vi "JSON GRUPO 2.vi"(8 "error in":errorcluster, 11 "Grupo in":T1(array[cluster])) -> (0 "error out":errorcluster, 1 "alarmas":refnum<class "JSON Array.lvclass">[](array[class]), 2 "JSON BAT":refnum<class "JSON Object.lvclass">[](array[class]), 3 "JSON CARGA":refnum<class "JSON Array.lvclass">[](array[class]), 5 "JSON FV":refnum<class "JSON Object.lvclass">[](array[class]))   [LabVIEW 2015]
uses:
  <vilib>/addons/JSON API/JSON Scalar/Set SGL.vi
  <vilib>/addons/JSON API/JSON Scalar/Set U32.vi
  <vilib>/addons/JSON API/JSON Object/JSON Object.lvclass
  <vilib>/addons/JSON API/JSON Array/JSON Array.lvclass
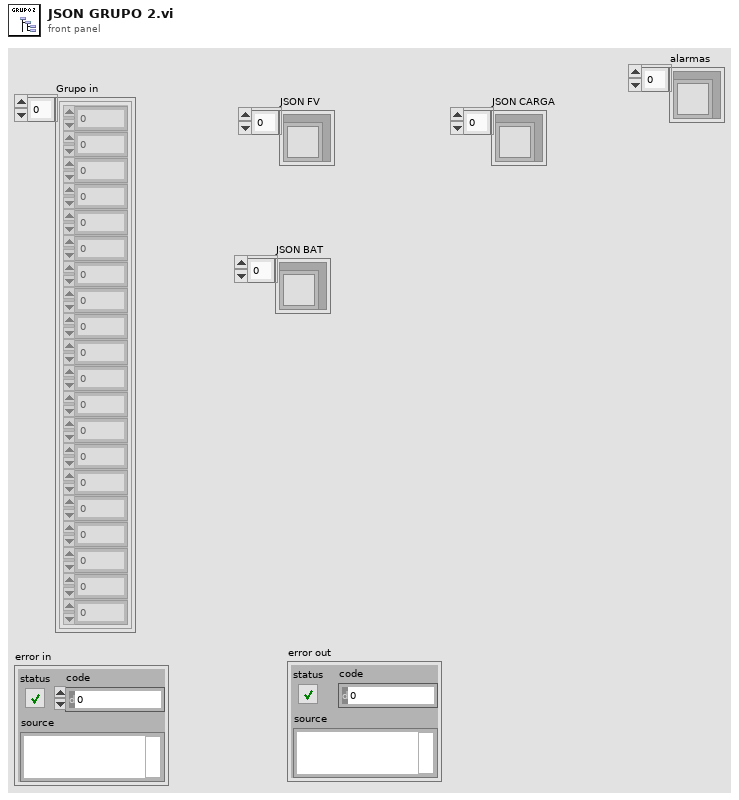
[diagram p1: front panel]
types:
  T1 = cluster{u32, dbl, dbl, dbl, dbl, dbl, dbl, dbl, dbl, dbl, dbl, dbl, dbl, dbl, dbl, dbl, dbl, dbl, dbl, dbl}[]
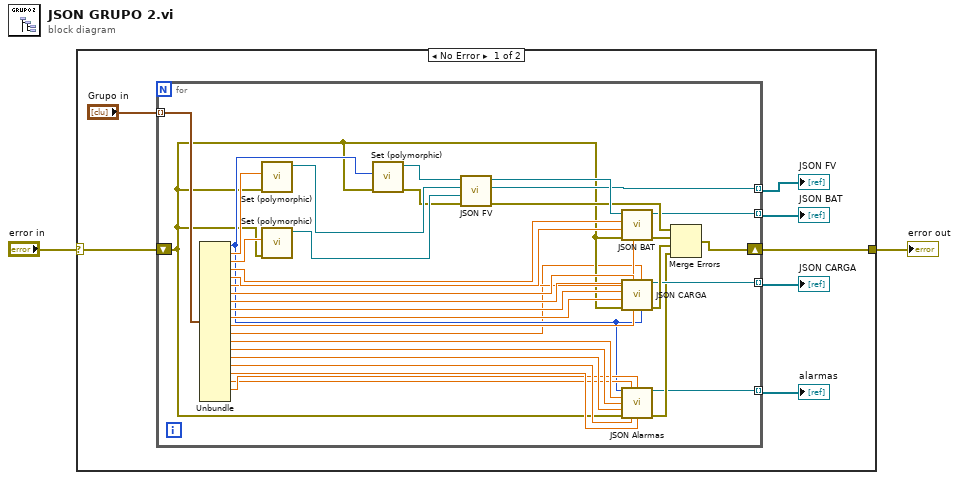
[diagram p0: block diagram]
diagram:
  n1 = case shown="No Error" "error in" {
    selector: "error in" -> [w3 w45]
    tunnel: [w4 w45] -> w1
    frame No Error {
      n2 = for {
        tunnel: "Grupo in" -> [w44] mode=indexing
        tunnel: [w28] -> w6 mode=indexing
        tunnel: [w27] -> w7 mode=indexing
        tunnel: [w26] -> w8 mode=indexing
        tunnel: [w13] -> w5 mode=indexing
        shift-right: [w12] -> w4
        shift-left: w3 -> [w11]
        n3 = Unbundle(w44) -> (w15:u32, w42:dbl, w41:dbl, w40:dbl, w37:dbl, w32:dbl, w34:dbl, w33:dbl, w25:dbl, w24:dbl, w23:dbl, w10:dbl, w22:dbl, w21:dbl, w20:dbl, w19:dbl, w18:dbl, w16:dbl, w17:dbl)  [unwired: 1 out]
        n4 = call-poly <vilib>:"Set (polymorphic).vi"("error in (no error)"=w11, "Numeric"=w42) -> ("JSON Scalar out"=w39:refnum<class "JSON Scalar.lvclass">)  [unwired: 8 in, 1 out]
        n5 = call-poly <vilib>:"Set (polymorphic).vi"("error in (no error)"=w11, "Numeric"=w41) -> ("JSON Scalar out"=w38:refnum<class "JSON Scalar.lvclass">)  [unwired: 8 in, 1 out]
        n6 = call-poly <vilib>:"Set (polymorphic).vi"("error in (no error)"=w11, "Numeric"=w15) -> ("error out"=w36:errorcluster, "JSON Scalar out"=w43:refnum<class "JSON Scalar.lvclass">)  [unwired: 8 in]
        n7 = call "JSON FV.vi"("error in"=w36, "JSON Scalar in 3"=w38, "JSON Scalar in 2"=w39, "JSON Scalar in 1"=w43) -> ("error out"=w31:errorcluster, "JSON Object out"=w26:refnum<class "JSON Object.lvclass">, "Instante"=w35:refnum<class "JSON Object.lvclass">)  [unwired: 5 in]
        n8 = call "JSON BAT.vi"("Numeric"=w32, "error in"=w11, "Numeric 2"=w37, "Numeric 3"=w40, "JSON Object in"=w35) -> ("error out"=w30:errorcluster, "JSON Object out"=w27:refnum<class "JSON Object.lvclass">)  [unwired: 5 in]
        n9 = call "JSON CARGA.vi"("time"=w15, "Potencia Fase 3"=w10, "Corriente Fase 3"=w23, "Corriente Fase 1"=w34, "error in"=w11, "Potencia Fase 2"=w24, "Corriente Fase 2"=w25, "Potencia Fase 1"=w33) -> ("error out"=w29:errorcluster, "JSON Array out"=w28:refnum<class "JSON Array.lvclass">)  [unwired: 2 in]
        n10 = call "JSON Alarmas.vi"("time"=w15, "high bat"=w16, "Fault Modul"=w17, "Temperatura"=w22, "Common Sys"=w21, "out line 1"=w20, "error in"=w11, "out line 3"=w19, "low bat"=w18) -> ("alarmas"=w13:refnum<class "JSON Array.lvclass">, "error out"=w14:errorcluster)  [unwired: 5 in]
        n11 = Merge Errors(w31, w30, w29, w14) -> (w12:errorcluster)
      }
      "JSON FV" <- w8
      "JSON BAT" <- w7
      "JSON CARGA" <- w6
      "alarmas" <- w5
    }
    frame Error {
    }
  }
  "error out" <- w1
